vi "analogtriger.vi"() -> ()   [LabVIEW 2018]
uses:
  <vilib>/rvi/Emulation/niFpgaGetClockAttributes.vi
  <vilib>/rvi/Emulation/niFpgaSctlEmulationGetInTimedLoop.vi
  <vilib>/rvi/Emulation/niFpgaEmulationReportErrorSimple.vi
  <vilib>/rvi/eio/common/nirviEmuTemplateMethod_errors.vi
  <vilib>/rvi/Emulation/niFpgaCriticalErrorInLSC.vi
  <vilib>/eio/EIONode/EIONode.xnode
panel:
  out "A/AI1":bool
  in  "Lower Threshold":u16=150
  in  "Sample rate (Ticks)":u32=80
  out "Loop Timer":u32
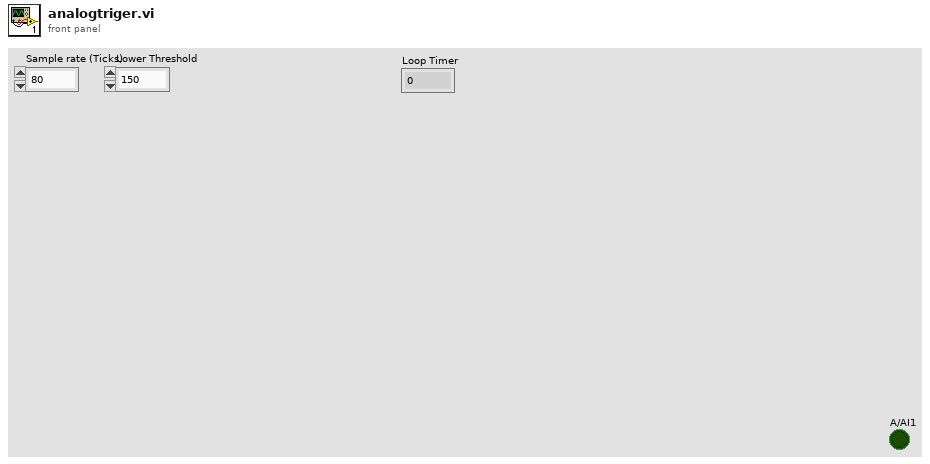
[diagram p1: front panel]
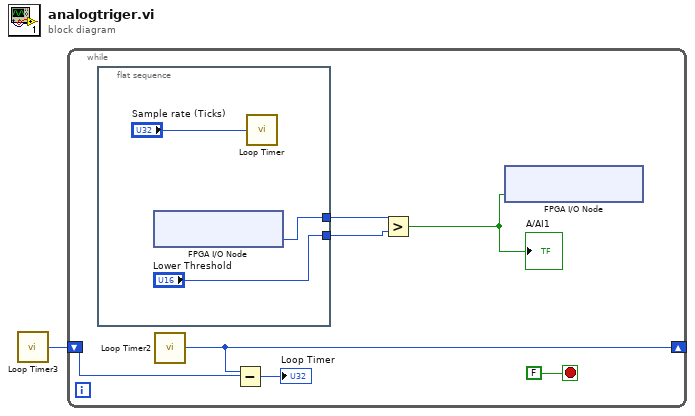
[diagram p0: block diagram]
diagram:
  n1 = call "Loop Timer3"() -> ("Tick Count(Ticks)"=w1:u32)  [unwired: 1 in]
  n2 = while {
    shift-right: [w7] -> _
    shift-left: w1 -> [w6]
    stop <- FALSE stop-if-true
    n3 = flat-sequence {
      tunnel: ["Lower Threshold"] -> w3
      tunnel: [w9] -> w4
      frame #0 {
        n4 = xnode "FPGA I/O Node"() -> ("ConnectorA/AI1"=w9:u16)  [unwired: 1 in, 1 out]
        n5 = call "Loop Timer"("Count(Ticks)"="Sample rate (Ticks)") -> ()  [unwired: 1 out]
      }
    }
    n6 = call "Loop Timer2"() -> ("Tick Count(Ticks)"=w7:u32)  [unwired: 1 in]
    n7 = Subtract(x=w7, y=w6) -> (x-y=→"Loop Timer":u32)
    n8 = Greater?(x=w4, y=w3) -> (0:w2:bool)
    "A/AI1" <- w2
    n9 = xnode "FPGA I/O Node"("ConnectorA/DIO1"=w2) -> ()  [unwired: 1 in, 1 out]
  }
